vi "coordinateArray.vi"(1 "width of represented x (or y) range (in m; default 1E-3=1mm)":sgl=0.001 format="%.2p", 2 "array size (default 64)":i32=64) -> (0 "x array":sgl[](array[numeric]) format="%.2f")   [LabVIEW 2024]
panel:
  # "width"
  # "index:"
  # "0"
  # "N-1"
  # "N"
  # "x"
  # "x value:"
  # "0"
  # "(note:  delta_x = distance between neighbouring elements\n= (width of represented range)/(array size)"
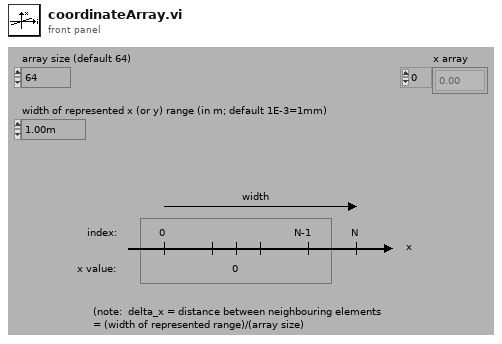
[diagram p1: front panel]
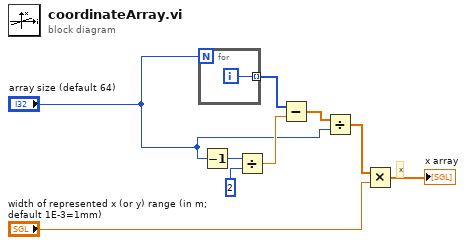
[diagram p0: block diagram]
diagram:
  # "x"
  n1 = for {
    N: "array size (default 64)" -> [_]
    tunnel: [w10] -> w7 mode=indexing
    i -> [w10]
  }
  n2 = Decrement(x="array size (default 64)") -> (x-1=w1:i32)
  n3 = Divide(x=w1, y=2) -> (x/y=w8:dbl)
  n4 = Subtract(x=w7, y=w8) -> (x-y=w6:dbl[])
  n5 = Divide(x=w6, y="array size (default 64)") -> (x/y=w5:dbl[])
  n6 = Multiply(x=w5, y="width of represented x (or y) range (in m; default 1E-3=1mm)") -> (x*y=→"x array":dbl[])
